vi "Status.get.vi"(8 "error in (no error)":errorcluster, 11 "EventDaemon in":refnum<class "ErrorDaemon.lvclass">) -> (0 "error out":errorcluster, 2 "current status":T1, 3 "EventDaemon out":refnum<class "ErrorDaemon.lvclass">)   [LabVIEW 2020, in "ErrorDaemon.lvclass"]
uses:
  ErrorDaemon.lvclass
  status--cluster.ctl
  states--enum.ctl
  ErrorDaemon.lvclass/ErrorDaemon.ctl
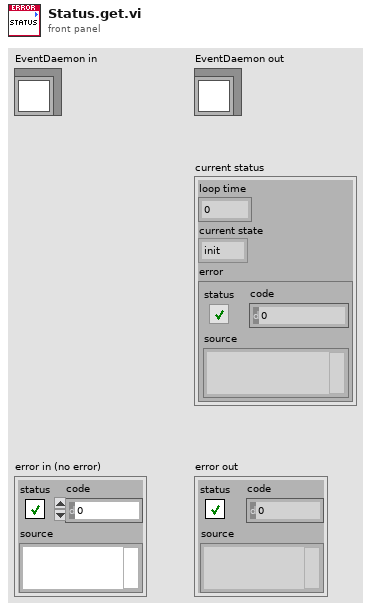
[diagram p1: front panel]
types:
  T1 = typedef "ErrorDaemon.lvclass/status--cluster.ctl" = cluster{"loop time":u32, "current state":T2, "error":errorcluster}
  T2 = typedef "ErrorDaemon.lvclass/states--enum.ctl" = enum16{"init", "default", "error handler", "exit"}
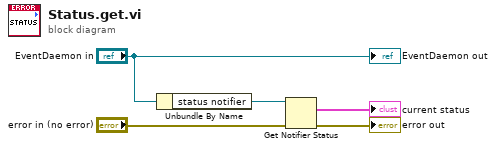
[diagram p0: block diagram]
diagram:
  n1 = Unbundle By Name("EventDaemon in") -> ("status notifier"=w5:refnum<notifier>)
  n2 = Get Notifier Status(notifier=w5, error in (no error)="error in (no error)") -> (current notification=→"current status":T1, error out=→"error out":errorcluster)  [unwired: 3 out]
  "EventDaemon out" <- "EventDaemon in"
